vi "GPIB_logging_multi-channel.vi"() -> ()   [LabVIEW 2018]
panel:
  out "error out":errorcluster
  out "Temperature (K)":string
  in  "Temperature":enum32{"Read Temperature", "Read Resistance"}(radio)
  in  "PID setting":string(combo)
  out "Controller Temp(K)":sgl format="%#_4g"
  in  "Channel":dbl=5.0
  in  "Controller":bool
  in  "Plot":bool
  in  "Set point (K)":dbl
  in  "Rate (K/s)":dbl=0.001
  in  "D:":string="50"
  in  "I:":string="10"
  in  "P:":string="2"
  in  "Ramp":bool
  in  "Controller address":string="3"
  in  "Sampling rate (ms)":u32=1000
  out "Time (s)":u32
  out "Controller temperature":cluster{"Y":dbl[], "Y":dbl[]}[](graph)
  in  "Record":bool
  in  "Start":bool
  in  "Stop program":bool
  in  "Data address":string="4"
  out "Reading error":errorcluster
  out "Resistance (Ohm)":string
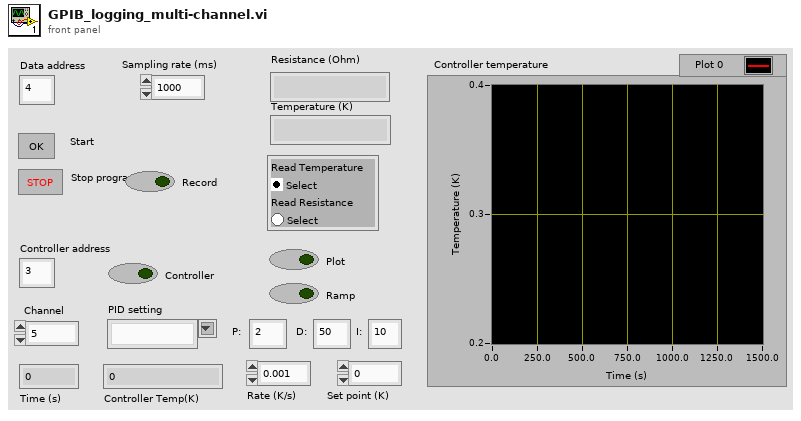
[diagram p1: front panel]
types:
  T1 = enum16{"open", "replace", "create", "open or create", "replace or create", "replace or create with confirmation"}
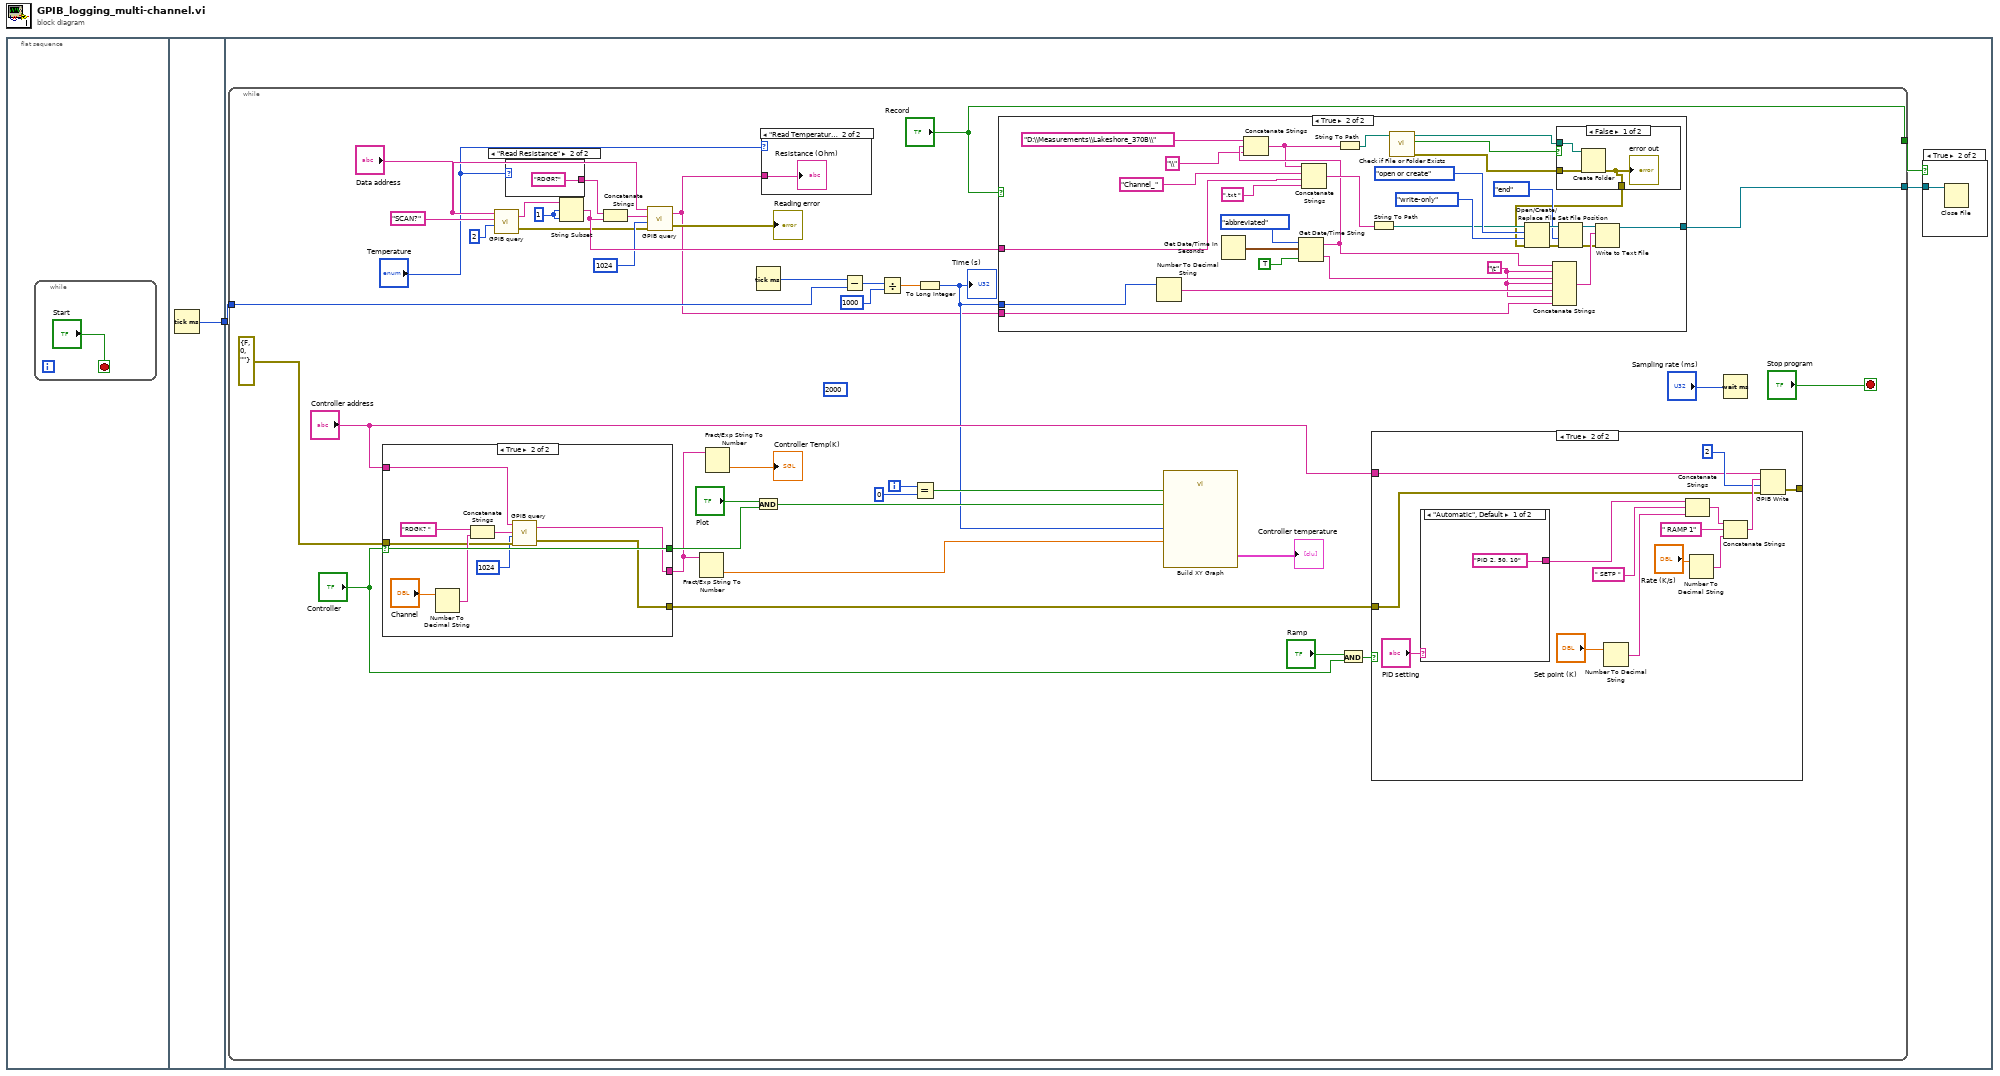
[diagram p0: block diagram]
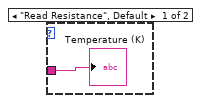
[diagram p3: hidden frame]
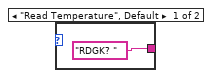
[diagram p4: hidden frame]
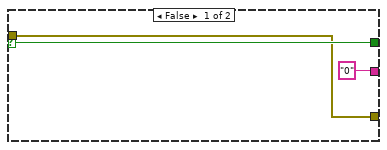
[diagram p5: hidden frame]
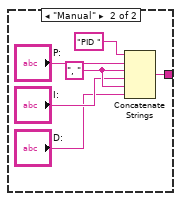
[diagram p7: hidden frame]
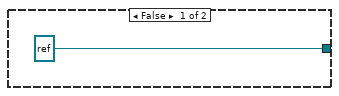
[diagram p8: hidden frame]
diagram:
  n1 = flat-sequence {
    tunnel: [w3] -> w1
    tunnel: w1 -> [w4]
    frame #0 {
      n2 = while {
        stop <- "Start" stop-if-true
      }
    }
    frame #1 {
      n3 = Tick Count (ms)() -> (millisecond timer value=w3:u32)
    }
    frame #2 {
      n4 = while {
        tunnel: [w35] -> w6
        tunnel: ["Record"] -> w5
        tunnel: w4 -> [w43]
        i -> [w27]
        stop <- "Stop program" stop-if-true
        w36 = 1 ("offset (0)")
        (unwired) 2000 ("timeout ms (488.2 global)")
        n5 = case shown="True" "Controller" {
          selector: "Controller" -> [w53 w63]
          tunnel: ["0" ("data") w55] -> w29
          tunnel: "Controller address" -> [_ w58]
          tunnel: errorcluster {"status"=FALSE, "code"=0, "source"=""} ("error in") -> [w52 w56]
          tunnel: [w53 w63] -> w30
          tunnel: [w52 w57] -> w22
          frame False {
          }
          frame True {
            n6 = Number To Decimal String(number="Channel") -> (decimal integer string=w60:string)  [unwired: 1 in]
            n7 = Concatenate Strings("RDGK? " ("data"), w60) -> (w59:string)
            n8 = call "GPIB query.vi"("address string"=w58, "data"=w59, "byte count"=1024, "error in"=w56) -> ("data 2"=w55:string, "error out (read)"=w57:errorcluster)  [unwired: 1 in]
          }
        }
        n9 = call "GPIB query.vi"("address string"="Data address", "data"="SCAN?", "byte count"=2) -> ("data 2"=w17:string, "error out (read)"=w9:errorcluster)  [unwired: 2 in]
        n10 = case shown="\"Read Resistance\"" "Temperature" {
          tunnel: ["RDGK? " ("command") "RDGR?" ("command")] -> w37
          frame "Read Temperature", Default {
          }
          frame "Read Resistance" {
          }
        }
        n11 = String Subset(string=w17, offset (0)=w36, length (rest)=w36) -> (substring=w16:string)
        n12 = Concatenate Strings(w37, w16) -> (w15:string)
        n13 = call "GPIB query.vi"("address string"="Data address", "data"=w15, "byte count"=1024, "error in"=w9) -> ("data 2"=w13:string, "error out (read)"=→"Reading error":errorcluster)  [unwired: 1 in]
        n14 = Fract/Exp String To Number(string=w29) -> (number=w44:dbl)  [unwired: 3 in, 1 out]
        n15 = Fract/Exp String To Number(string=w29) -> (number=→"Controller Temp(K)":dbl)  [unwired: 3 in, 1 out]
        n16 = Tick Count (ms)() -> (millisecond timer value=w34:u32)
        n17 = And(x="Plot", y=w30) -> (x .and. y?=w32:bool)
        n18 = case shown="\"Read Temperature\"" "Temperature" {
          tunnel: w13 -> [w47 w48]
          frame "Read Resistance", Default {
            "Temperature (K)" <- w47
          }
          frame "Read Temperature" {
            "Resistance (Ohm)" <- w48
          }
        }
        n19 = Subtract(x=w34, y=w43) -> (x-y=w42:u32)
        n20 = Divide(x=w42, y=u32 1000) -> (x/y=w41:dbl)
        n21 = Equal?(x=w27, y=0) -> (x = y?=w25:bool)
        n22 = To Long Integer(number=w41) -> (32bit integer=w23:i32)
        "Time (s)" <- w23
        n23 = case shown="True" "Record" {
          tunnel: [refnum<file> refnum ("refnum out") w117] -> w35
          tunnel: w23 -> [_ w116]
          tunnel: w16 -> [_ w100]
          tunnel: w13 -> [_ w111]
          frame False {
          }
          frame True {
            w107 = "\t"
            n24 = Number To Decimal String(number=w116) -> (decimal integer string=w108:string)  [unwired: 1 in]
            n25 = Get Date/Time In Seconds() -> (seconds since 1Jan1904=w112:timestamp)
            n26 = Get Date/Time String(date format (0)=enum16{"short", "long", "abbreviated"}."abbreviated", seconds (now)=w112, want seconds? (F)=TRUE) -> (date string=w94:string, time string=w114:string)
            n27 = Concatenate Strings("D:\\Measurements\\Lakeshore_370B\\" ("string"), w94, "\\" ("string")) -> (w91:string)
            n28 = Concatenate Strings(w91, "Channel_", w100, ".txt ") -> (w98:string)
            n29 = String To Path(string=w91) -> (path=w92:path)
            n30 = String To Path(string=w98) -> (path=w97:path)
            n31 = call <vilib>:"Check if File or Folder Exists.vi"("path"=w92) -> ("error out"=w88:errorcluster, "file or folder exists?"=w90:bool, "dup path"=w89:path)  [unwired: 8 in]
            n32 = Concatenate Strings(w94, w107, w114, w107, w108, w107, w111) -> (w109:string)
            n33 = case shown="False" w90 {
              tunnel: w89 -> [w120 _]
              tunnel: w88 -> [w119 w121]
              tunnel: [w118 w121] -> w87
              frame False {
                n34 = Create Folder(path (use dialog)=w120, error in=w119) -> (error out=w118:errorcluster)  [unwired: 1 in, 2 out]
                "error out" <- w118
              }
              frame True {
              }
            }
            n35 = Open/Create/Replace File(file path (use dialog)=w97, error in=w87, operation (0:open)=T1."open or create", access (0:read/write)=enum16{"read/write", "read-only", "write-only"}."write-only") -> (refnum out=w106:refnum<file>, error out=w105:errorcluster)  [unwired: 2 in, 1 out]
            n36 = Set File Position(refnum=w106, from (0:start)=enum16{"start", "end", "current"}."end", error in=w105) -> (refnum out=w103:refnum<file>, error out=w104:errorcluster)  [unwired: 1 in]
            n37 = Write to Text File(file (use dialog)=w103, text=w109, error in=w104) -> (refnum out=w117:refnum<file>)  [unwired: 1 in, 2 out]
          }
        }
        n38 = call "Build XY Graph"("Enable"=w32, "Reset"=w25, "Y Input"=w44, "X Input"=w23) -> ("XY Graph"=→"Controller temperature":cluster{"X":dbl[], "Y":dbl[]}[])  [unwired: 6 in, 1 out]
        n39 = And(x="Ramp", y="Controller") -> (x .and. y?=w20:bool)
        n40 = case shown="True" w20 {
          tunnel: "Controller address" -> [_ w72]
          tunnel: [w64 w71] -> _
          tunnel: w22 -> [w64 w66]
          frame False {
          }
          frame True {
            n41 = case shown="\"Automatic\", Default" "PID setting" {
              tunnel: ["PID 2, 50, 10" w80] -> w76
              frame "Automatic", Default {
              }
              frame "Manual" {
                w83 = ", " ("string")
                n42 = Concatenate Strings("PID " ("string"), "P:", w83, "I:", w83, "D:") -> (w80:string)
              }
            }
            n43 = Number To Decimal String(number="Set point (K)") -> (decimal integer string=w69:string)  [unwired: 1 in]
            n44 = Concatenate Strings(w76, " SETP " ("data"), w69) -> (w74:string)
            n45 = Number To Decimal String(number="Rate (K/s)") -> (decimal integer string=w67:string)  [unwired: 1 in]
            n46 = Concatenate Strings(w74, " RAMP 1" ("data"), w67) -> (w77:string)
            n47 = GPIB Write(0:w72, 1:w77, 2:i16 2 ("mode (0)"), 3:w66) -> (6:w71:errorcluster)  [unwired: 1 in, 1 out]
          }
        }
        n48 = Wait (ms)(milliseconds to wait="Sampling rate (ms)") -> ()  [unwired: 1 out]
      }
      n49 = case shown="True" w5 {
        tunnel: w6 -> [_ w7]
        frame False {
        }
        frame True {
          n50 = Close File(refnum=w7) -> ()  [unwired: 1 in, 2 out]
        }
      }
    }
  }
